vi "create server acceptor.vi"(8 "error in":errorcluster, 9 "port":u16, 11 "engine":u64) -> (0 "error out":errorcluster, 3 "acceptor out":u64)   [LabVIEW 2016, in "async tls dl.lvlib"]
uses:
  async tls dl.lvlib
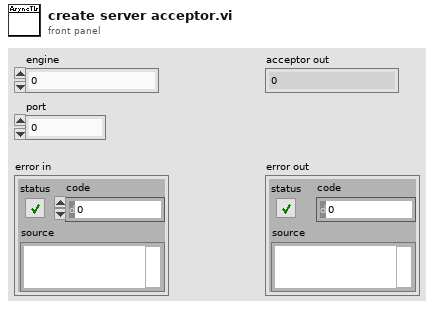
[diagram p1: front panel]
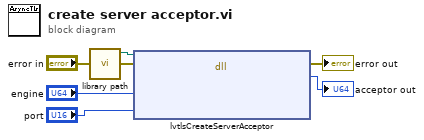
[diagram p0: block diagram]
diagram:
  n1 = call "library path.vi"() -> ("path"=w1:path)  [unwired: 11 in]
  n2 = dll-call lib="C:/Users/IEUser/Desktop/libasynclvtls/lvasynctls.dll" fn="lvtlsCreateServerAcceptor"(path in=w1, error in="error in", "engine"="engine", "port"="port") -> (error out=→"error out":errorcluster, "acceptor"=→"acceptor out":u64)  [unwired: 3 in, 1 out]
